vi "Create I2C Devices.vi"(8 "error in (no error)":errorcluster, 11 "Driver Test in":refnum<class "Driver Test.lvclass">) -> (0 "error out":errorcluster, 3 "I2C Devices":refnum<class "NI-8451.lvclass">[](array[class]))   [LabVIEW 2015, in "Driver Test.lvclass"]
doc: "Creates an I2C device for each active position."
uses:
  Driver Test.lvclass
  Classes/Instruments/I2C Device/NI-8451/NI-8451.lvclass
  <vilib>/Cree, Inc/Cree Test Framework/Classes/Base Objects/Base Class/Base Class/Base Class.lvclass
  Classes/Instruments/I2C Device/I2C Device/Class/I2C Device.lvclass
  Test Class/Test Class.lvclass
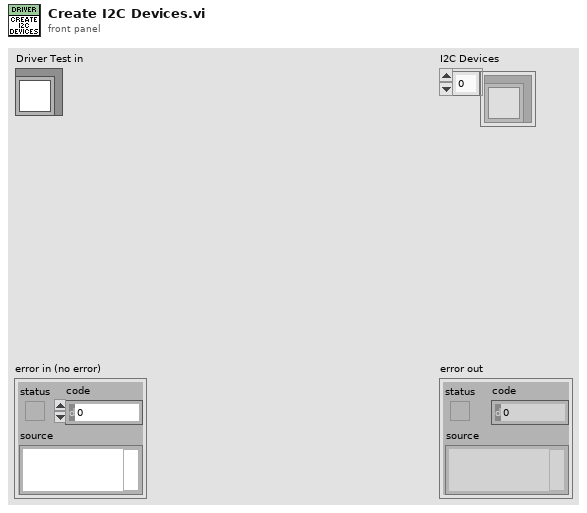
[diagram p1: front panel]
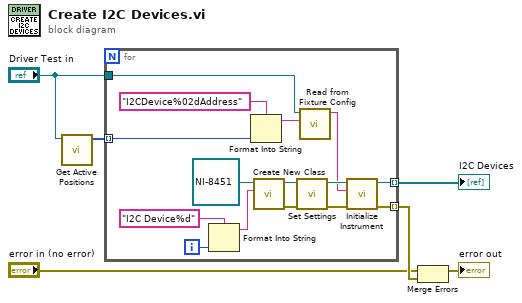
[diagram p0: block diagram]
diagram:
  n1 = call "Get Active Positions.vi"("Test Class in"="Driver Test in") -> ("Active Positions"=w2:u32[])  [unwired: 9 in, 1 out]
  n2 = for {
    tunnel: w2 -> [w21] mode=indexing
    tunnel: "Driver Test in" -> [w7]
    tunnel: [w14] -> w5 mode=indexing
    tunnel: [w13] -> w6 mode=indexing
    i -> [w12]
    n3 = Format Into String(format string="I2C Device%d", w12) -> (resulting string=w11:string)  [unwired: 2 in, 1 out]
    n4 = Format Into String(format string="I2CDevice%02dAddress", w21) -> (resulting string=w9:string)  [unwired: 2 in, 1 out]
    n5 = call <vilib>:"Create New Class.vi"("Name"=w11, "Base Class in"=refnum<class "NI-8451.lvclass"> refnum ("NI-8451.lvlib:NI-8451.lvclass")) -> ("error out"=w16:errorcluster, "Base Class out"=w18:refnum<class "NI-8451.lvclass">)  [unwired: 8 in]
    n6 = call "Set Settings.vi"("error in (no error)"=w16, "Acrobat Template in"=w18) -> ("error out"=w15:errorcluster, "Acrobat Template out"=w17:refnum<class "NI-8451.lvclass">)  [unwired: 8 in]
    n7 = call-dynamic "Read from Fixture Config.vi"("Key"=w9, "Test Class in"=w7) -> ("Instrument Info"=w8:string)  [unwired: 8 in, 1 out]
    n8 = call-dynamic "Initialize Instrument.vi"("error in (no error)"=w15, "Instrument Address"=w8, "Acrobat Template in"=w17) -> ("error out"=w13:errorcluster, "Acrobat Template out"=w14:refnum<class "NI-8451.lvclass">)  [unwired: 7 in]
  }
  "I2C Devices" <- w5
  n9 = Merge Errors("error in (no error)", w6) -> (→"error out":errorcluster)
